vi "matlab-for-complementary-filter1.vi"() -> ()   [LabVIEW 2016]
panel:
  out "Path Length":dbl
  in  "Acceleration Data (g)":T1
  in  "Gyro  Data (dps)":T1
  out "angle_y":dbl
  out "angle_x":dbl
  out "error out":errorcluster
  in  "error in (no error)":errorcluster
  out "x_pos":dbl
  out "y_pos":dbl
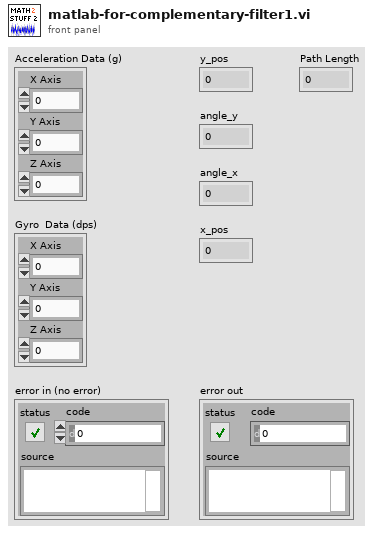
[diagram p1: front panel]
types:
  T1 = cluster{"X Axis":i16, "Y Axis":i16, "Z Axis":i16}
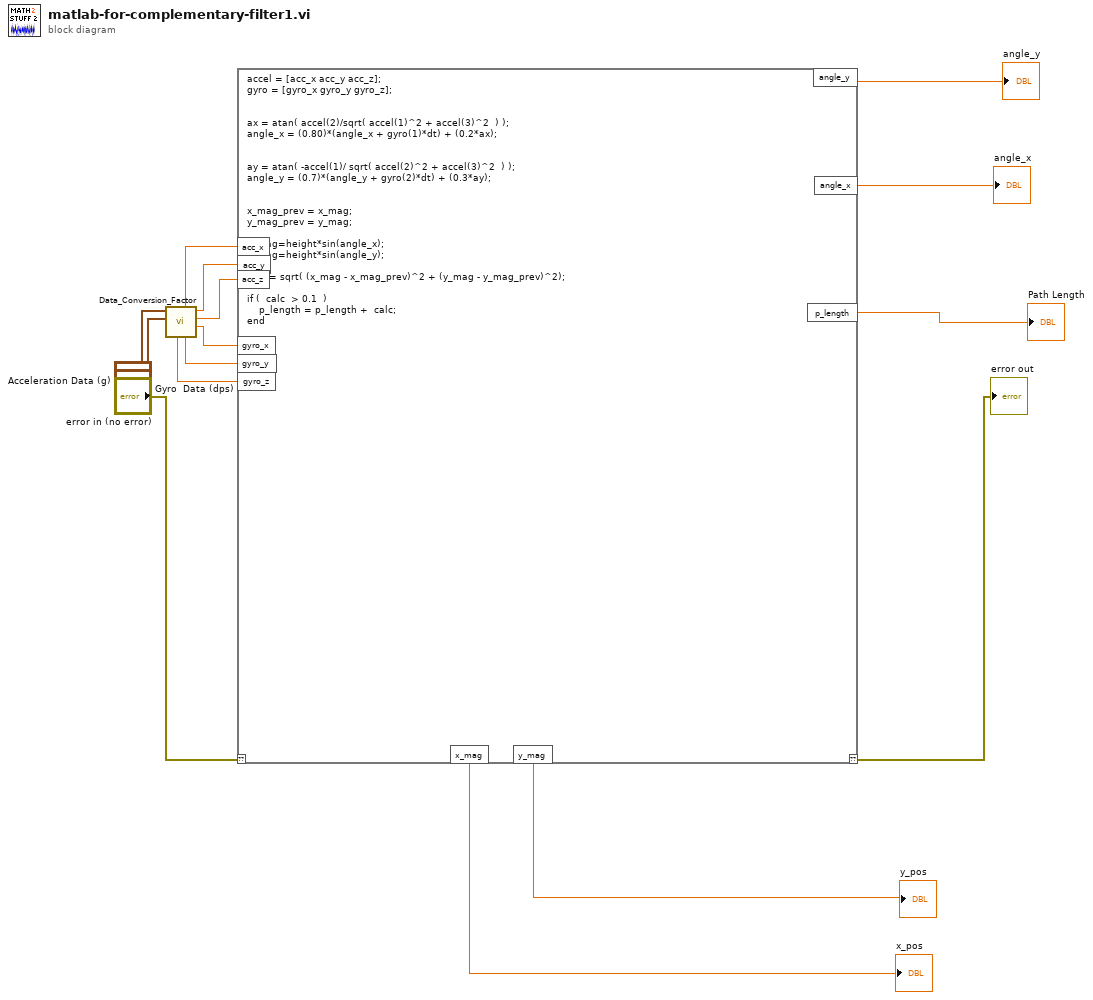
[diagram p0: block diagram]
diagram:
  n1 = call "Data_Conversion_Factor.vi"("Gyro  Data (dps)"="Gyro  Data (dps)", "Acceleration Data (g)"="Acceleration Data (g)") -> ("Gyro_X"=w10:dbl, "Accel_Z"=w9:dbl, "Accel_Y"=w8:dbl, "Gyro_Y"=w11:dbl, "Accel_X"=w7:dbl, "Gyro_Z"=w12:dbl)  [unwired: 4 in]
  n2 = script code="accel = [acc_x acc_y acc_z];\ngyro = [gyro_x gyro_y gyro_z];\n\n\nax = atan( accel(2)/sqrt( accel(1)^2 + accel(3)^2  ) );\nangle_x = (0.80)*(angle_x + gyro(1)*dt) + (0.2*ax);\n\n\nay = atan( -accel(1)/ sqrt( accel(2)^2 + accel(3)^2  ) );\nangle_y = (0.7)*(angle_y + gyro(2)*dt) + (0.3*ay);\n\n\nx_mag_prev = x_mag;\ny_mag_prev = y_mag;\n\nx_mag=height*sin(angle_x); \ny_mag=height*sin(angle_y); \n\ncalc = sqrt( (x_mag - x_mag_prev)^2 + (y_mag - y_mag_prev)^2);\n\nif (  calc  > 0.1  ) \n    p_length = p_length +  calc;\nend"("??"="error in (no error)", "acc_y"=w8, "acc_z"=w9, "gyro_x"=w10, "gyro_y"=w11, "gyro_z"=w12, "acc_x"=w7) -> ("??"=→"error out":errorcluster, "angle_y"=→"angle_y":dbl, "angle_x"=→"angle_x":dbl, "x_mag"=→"x_pos":dbl, "y_mag"=→"y_pos":dbl, "p_length"=→"Path Length":dbl)
